vi "Numeric, Timestamp, and DBL from TDMS.vi"(8 "error in (no error)":errorcluster, 9 "Group and Tracks":T3, 10 "Graph Samples":T1={"Start"="", "Max Samples"=30, "End"=""} {"Max Samples" min=1}, 11 "Refnum in":refnum<k34>) -> (0 "error out":errorcluster, 2 "Numeric, Timestamp, and DBL from TDML":T2, 3 "Refnum out":refnum<k34>)   [LabVIEW 2023]
uses:
  <vilib>/gmath/NI_Gmath.lvlib
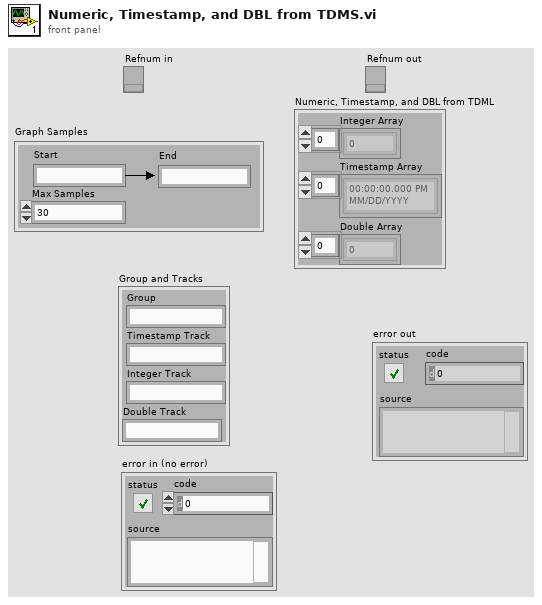
[diagram p1: front panel]
types:
  T1 = cluster{"Start":string, "Max Samples":u64, "End":string}
  T2 = cluster{"Integer Array":i32[], "Timestamp Array":timestamp[], "Double Array":dbl[]}
  T3 = cluster{"Group":string, "Timestamp Track":string, "Integer Track":string, "Double Track":string}
  T4 = cluster{"Numeric Array":i32[], "Timestamp Array":timestamp[], "DBL Array":dbl[]}
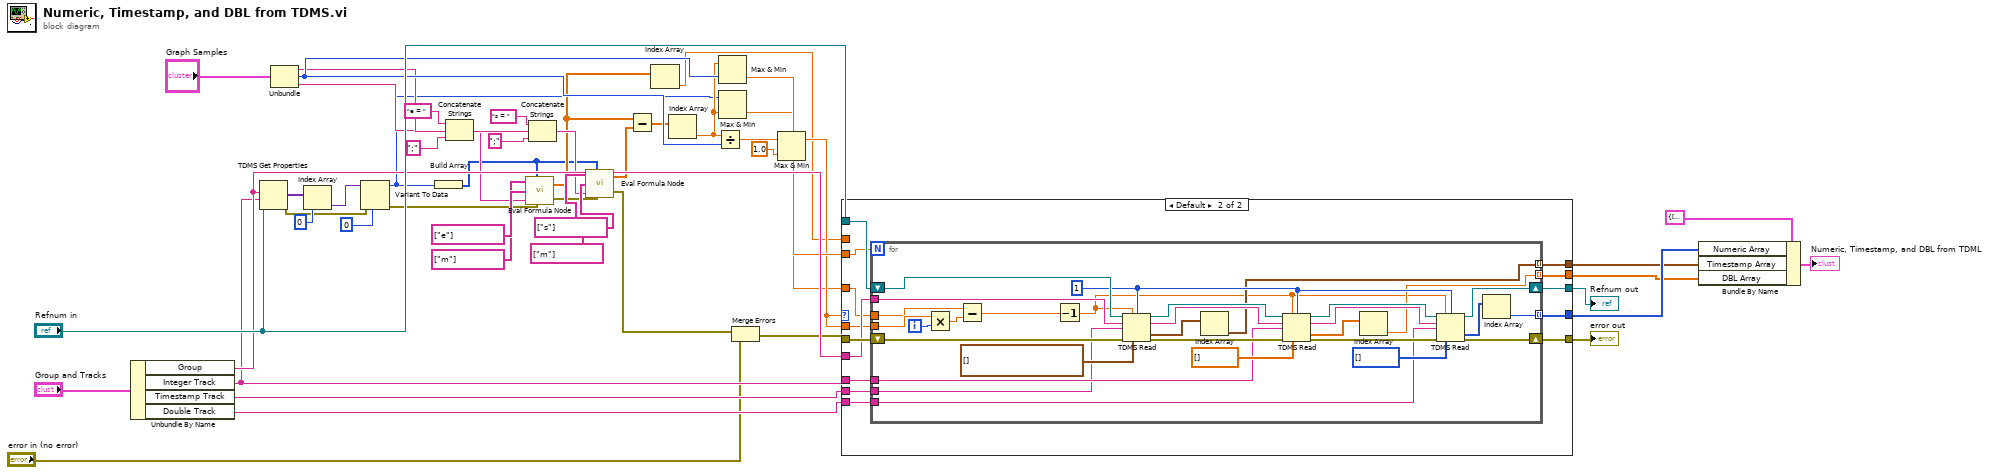
[diagram p0: block diagram]
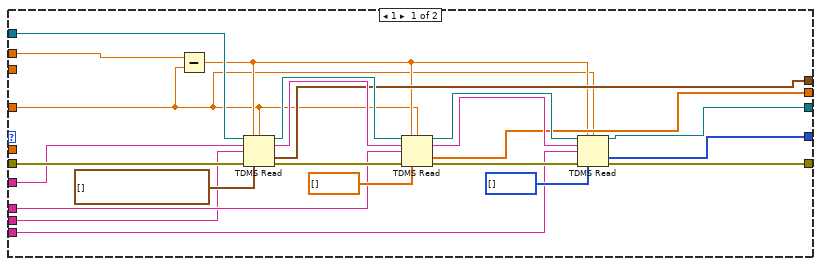
[diagram p2: hidden frame]
diagram:
  n1 = Unbundle By Name("Group and Tracks") -> ("Group"=w33:string, "Integer Track"=w32:string, "Timestamp Track"=w46:string, "Double Track"=w47:string)
  n2 = TDMS Get Properties(9:w32, 10:w33, 11:"Refnum in") -> (0:w4:errorcluster, 4:w29:variant[])  [unwired: 3 in, 4 out]
  n3 = Unbundle("Graph Samples") -> ("Start"=w22:string, "Max Samples"=w28:u64, "End"=w18:string)
  n4 = Index Array(array=w29, index=0) -> (element=w30:variant)
  n5 = Variant To Data(error in=w4, type=0, Variant=w30) -> (data=w7:i32, error out=w3:errorcluster)
  n6 = Build Array(w7) -> (w8:i32[])
  n7 = Concatenate Strings("e = " ("string"), w18, ";" ("string")) -> (w17:string)
  n8 = call <vilib>:"Eval Formula Node.vi"("Variables Input"=string[] ["m"], "Input Values"=w8, "Variables Output"=string[] ["e"], "formula"=w17, "error in (no error)"=w3) -> ("Output Values"=w12:dbl[], "error out"=w2:errorcluster)
  n9 = Concatenate Strings("s = " ("string"), w22, ";" ("string")) -> (w21:string)
  n10 = call <vilib>:"Eval Formula Node.vi"("Variables Input"=string[] ["m"], "Input Values"=w8, "Variables Output"=string[] ["s"], "formula"=w21, "error in (no error)"=w2) -> ("Output Values"=w14:dbl[], "error out"=w1:errorcluster)
  n11 = Subtract(x=w12, y=w14) -> (x-y=w27:dbl[])
  n12 = Index Array(array=w12) -> (element=w11:dbl)  [unwired: 1 in]
  n13 = Index Array(array=w27) -> (element=w9:dbl)  [unwired: 1 in]
  n14 = Divide(x=w9, y=w28) -> (x/y=w25:dbl)
  n15 = Max & Min(x=w9, y=w28) -> (min(x,y)=w26:dbl)  [unwired: 1 out]
  n16 = Max & Min(x=w7, y=w9) -> (min(x,y)=w10:dbl)  [unwired: 1 out]
  n17 = Merge Errors(w1, "error in (no error)") -> (w5:errorcluster)
  n18 = Max & Min(x=w25, y=1.0) -> (max(x,y)=w13:dbl)  [unwired: 1 out]
  n19 = case shown="Default" w13 {
    tunnel: [w63 w86] -> w49
    tunnel: w5 -> [w61 w85]
    tunnel: [w62 w84] -> w48
    tunnel: w47 -> [w60 w83]
    tunnel: w46 -> [w58 w82]
    tunnel: [w53 w81] -> w45
    tunnel: [w54 w80] -> w43
    tunnel: [w55 w79] -> w42
    tunnel: "Refnum in" -> [w56 w78]
    tunnel: w33 -> [w57 w77]
    tunnel: w32 -> [w59 w76]
    tunnel: w26 -> [_ w75]
    tunnel: w13 -> [_ w74]
    tunnel: w11 -> [w52 _]
    tunnel: w10 -> [w50 w73]
    frame 1 {
      n20 = Subtract(x=w52, y=w50) -> (x-y=w51:dbl)
      n21 = TDMS Read(0:w56, 1:w51, 2:w50, 5:w57, 7:w58, 11:w61, 12:timestamp[] []) -> (4:w68:refnum<k34>, 6:w69:string, 10:w55:timestamp[], 15:w65:errorcluster)  [unwired: 1 in, 2 out]
      n22 = TDMS Read(0:w68, 1:w51, 2:w50, 5:w69, 7:w59, 11:w65, 12:dbl[] []) -> (4:w70:refnum<k34>, 6:w71:string, 10:w54:dbl[], 15:w64:errorcluster)  [unwired: 1 in, 2 out]
      n23 = TDMS Read(0:w70, 1:w51, 2:w50, 5:w71, 7:w60, 11:w64, 12:i32[] []) -> (4:w63:refnum<k34>, 10:w53:i32[], 15:w62:errorcluster)  [unwired: 1 in, 3 out]
    }
    frame Default {
      n24 = for {
        N: w75 -> [_]
        tunnel: w77 -> [w103]
        tunnel: w76 -> [w102]
        tunnel: w83 -> [w101]
        tunnel: w82 -> [w100]
        tunnel: [w90] -> w81 mode=indexing
        tunnel: [w92] -> w80 mode=indexing
        tunnel: [w94] -> w79 mode=indexing
        shift-right: [w114] -> w86
        shift-left: w78 -> [w110]
        shift-right: [w104] -> w84
        shift-left: w85 -> [w107]
        tunnel: w74 -> [w98]
        tunnel: w73 -> [w87]
        i -> [w89]
        w96 = 1
        n25 = Multiply(x=w98, y=w89) -> (x*y=w97:dbl)
        n26 = Subtract(x=w87, y=w97) -> (x-y=w95:dbl)
        n27 = Decrement(x=w95) -> (x-1=w88:dbl)
        n28 = TDMS Read(0:w110, 1:w88, 2:w96, 5:w103, 7:w100, 11:w107, 12:timestamp[] []) -> (4:w111:refnum<k34>, 6:w112:string, 10:w99:timestamp[], 15:w106:errorcluster)  [unwired: 1 in, 2 out]
        n29 = Index Array(array=w99) -> (element=w94:timestamp)  [unwired: 1 in]
        n30 = TDMS Read(0:w111, 1:w88, 2:w96, 5:w112, 7:w102, 11:w106, 12:dbl[] []) -> (4:w113:refnum<k34>, 6:w115:string, 10:w93:dbl[], 15:w105:errorcluster)  [unwired: 1 in, 2 out]
        n31 = Index Array(array=w93) -> (element=w92:dbl)  [unwired: 1 in]
        n32 = TDMS Read(0:w113, 1:w88, 2:w96, 5:w115, 7:w101, 11:w105, 12:i32[] []) -> (4:w114:refnum<k34>, 10:w91:i32[], 15:w104:errorcluster)  [unwired: 1 in, 3 out]
        n33 = Index Array(array=w91) -> (element=w90:i32)  [unwired: 1 in]
      }
    }
  }
  "Refnum out" <- w49
  "error out" <- w48
  n34 = Bundle By Name(cluster=T4 {"Numeric Array"=[], "Timestamp Array"=[], "DBL Array"=[]} ("input cluster"), "Numeric Array"=w45, "Timestamp Array"=w42, "DBL Array"=w43) -> (→"Numeric, Timestamp, and DBL from TDML":T4)
